vi "Size of Data from TD__ogtk.vi"(8 "error in":errorcluster, 10 "Type Descriptor":T1) -> (0 "error out":errorcluster, 2 "Size of Data":i32)   [LabVIEW 2011]
doc: "Returns the size of data of the TD. \nThe VI will return the following bytes of the listed datatypes:\n<b>1 byte</b> - I8, U8, Enum U8, Boolean\n<b>2 bytes</b> - 16, U16, Enum U16 \n<b>4 bytes</b> - I32, U32, SGL, Enum U32, Refnum\n<b>8 bytes</b> - I64, U64, DBL, CSG, Enum U64 \n<b>16 bytes</b> - EXT, CDB\n<b>32 bytes</b> - CXT\n<b>-1</b> - String, Path, Array \n<b>Sum of Bytes</b> - Cluster, VI calls itself recursively"
uses:
  Type Descriptor__ogtk.ctl
panel:
  in  "for recursive call to self":refnum<vi>
  # "[OpenG VI Tags] ***Do Not Remove***"
  # "Size of Data from TD.vi\n\nReturns the data size of the type defined by the TD.  This vi calls itself recurs\n\nPlease visit http://www.OpenG.org to learn about the\nOpen Source LabVIEW software movement.\n\nNOTICE -- YOU MUST LEAVE THIS NOTICE IN PLACE.  PER THE TERMS OF THE LICENSE BELOW, YOU MAY SUBLICENSE THIS SOFTWARE \nIN ANY WAY THAT DOES NOT CONFLICT WITH THIS LICENSE.\n\n### BSD License (http://www.opensource.org/licenses/bsd-license.php) Begin ###\n \nCopyright (c) 2002, Jean-Pierre Drolet <drolet_jp@hotmail.com>\nCopyright (c) 2002-2006, Jim Kring <jim@jimkring.com>\n\nAll rights reserved.\n\nRedistribution and use in source and binary forms, with or without modification, are permitted provided that the following conditions are met:\n\n    * Redistributions of source code must retain the above copyright notice, this list of conditions and the following disclaimer.\n    * Redistributions in binary form must reproduce the above copyright notice, this list of conditions and the following disclaimer in the \n       documentation and/or other materials provided with the distribution.\n    * Neither the name of SciWare, James Kring, Inc., nor the names of its contributors may be used to endorse or promote products derived \n       from this software without specific prior written permission.\n\nTHIS SOFTWARE IS PROVIDED BY THE COPYRIGHT HOLDERS AND CONTRIBUTORS \"AS IS\" AND ANY EXPRESS OR IMPLIED WARRANTIES, \nINCLUDING, BUT NOT LIMITED TO, THE IMPLIED WARRANTIES OF MERCHANTABILITY AND FITNESS FOR A PARTICULAR PURPOSE ARE \nDISCLAIMED. IN NO EVENT SHALL THE COPYRIGHT OWNER OR CONTRIBUTORS BE LIABLE FOR ANY DIRECT, INDIRECT, INCIDENTAL,\n SPECIAL, EXEMPLARY, OR CONSEQUENTIAL DAMAGES (INCLUDING, BUT NOT LIMITED TO, PROCUREMENT OF SUBSTITUTE GOODS OR \nSERVICES; LOSS OF USE, DATA, OR PROFITS; OR BUSINESS INTERRUPTION) HOWEVER CAUSED AND ON ANY THEORY OF LIABILITY, \nWHETHER IN CONTRACT, STRICT LIABILITY, OR TORT (INCLUDING NEGLIGENCE OR OTHERWISE) ARISING IN ANY WAY OUT OF THE USE \nOF THIS SOFTWARE, EVEN IF ADVISED OF THE POSSIBILITY OF SUCH DAMAGE.\n\n### BSD License End ###"
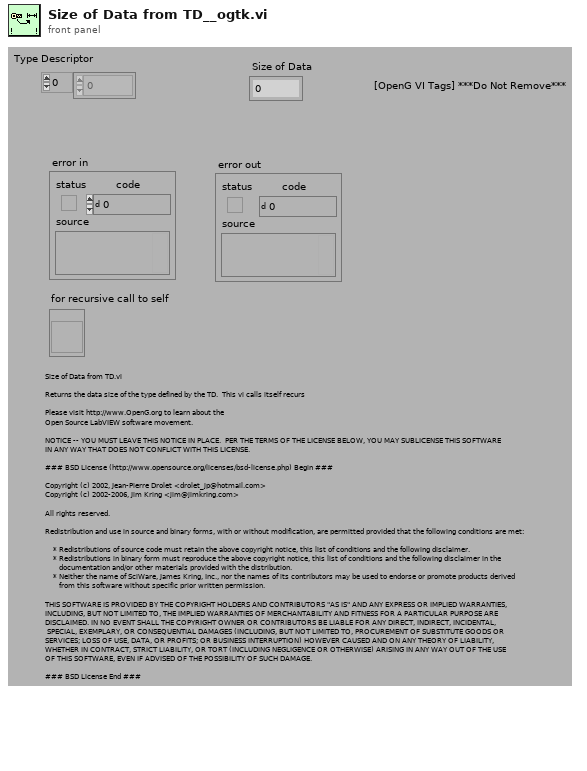
[diagram p1: front panel]
types:
  T1 = typedef "Type Descriptor__ogtk.ctl" = i16[]
  T2 = typedef "Type Descriptor Header__ogtk.ctl" = cluster{"length":u16, "private":u8, "type":T3, "# elements":u16}
  T3 = typedef "Type Descriptor Enumeration__ogtk.ctl" = enum8{"<Null>", "I8", "I16", "I32", "I64", "U8", "U16", "U32", "U64", "SGL", "DBL", "EXT", "CSG", "CDB", "CXT", "0x0F", "0x10", "0x11", "0x12", "0x13", "0x14", "Enum U8", "Enum U16", "Enum U32", "Enum U64", "SGL PQ", "DBL PQ", "EXT PQ", "CSG PQ", "CDB PQ", "CXT PQ", "0x1F", "0x20", "Boolean", "0x22", "0x23", "0x24", "0x25", "0x26", "0x27", "0x28", "0x29", "0x2A", "0x2B", "0x2C", "0x2D", "0x2E", "0x2F", "String", "0x31", "Path", "Pict", "0x34", "0x35", "0x36", "DAQ", "0x38", "0x39", "0x3A", "0x3B", "0x3C", "0x3D", "0x3E", "0x3F", "Array", "0x41", "0x42", "0x43", "0x44", "0x45", "0x46", "0x47", "0x48", "0x49", "0x4A", "0x4B", "0x4C", "0x4D", "0x4E", "0x4F", "Cluster", "0x51", "0x52", "Variant", "Waveform", "0x55", "0x56", "0x57", "0x58", "0x59", "0x5A", "0x5B", "0x5C", "0x5D", "0x5E", "0x5F", "0x60", "0x61", "0x62", "0x63", "0x64", "0x65", "0x66", "0x67", "0x68", "0x69", "0x6A", "0x6B", "0x6C", "0x6D", "0x6E", "0x6F", "Refnum"}
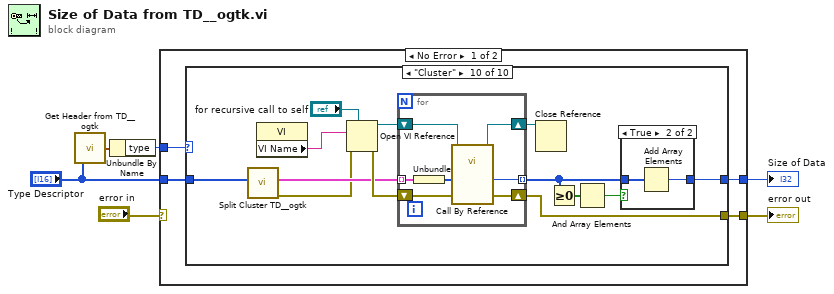
[diagram p0: block diagram]
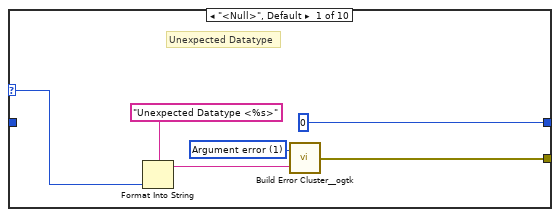
[diagram p2: hidden frame]
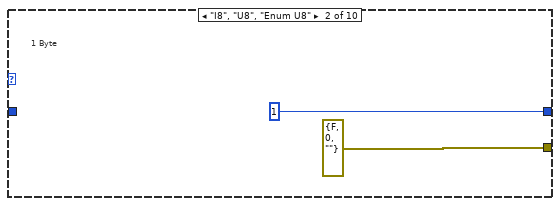
[diagram p3: hidden frame]
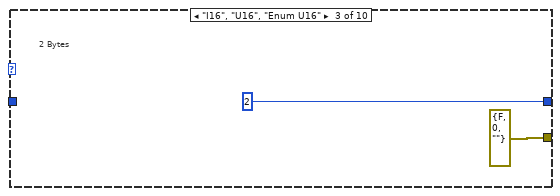
[diagram p4: hidden frame]
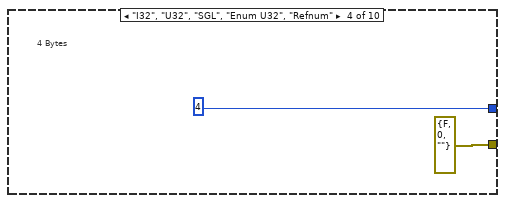
[diagram p5: hidden frame]
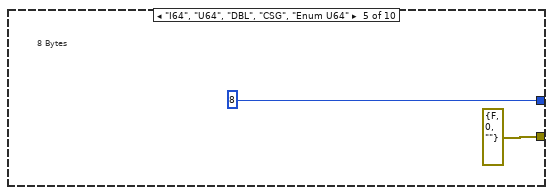
[diagram p6: hidden frame]
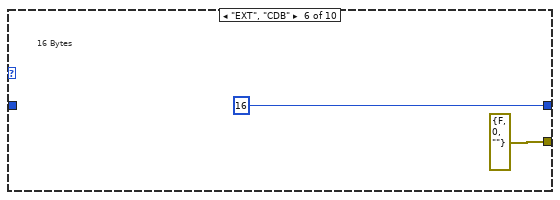
[diagram p7: hidden frame]
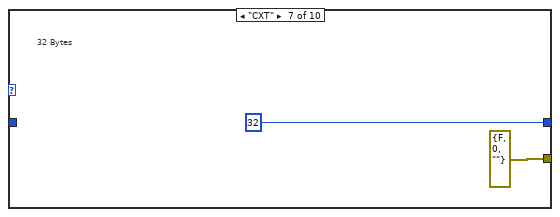
[diagram p8: hidden frame]
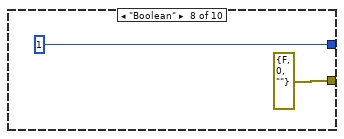
[diagram p9: hidden frame]
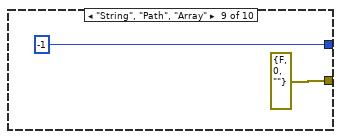
[diagram p10: hidden frame]
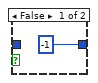
[diagram p11: hidden frame]
diagram:
  n1 = call "Get Header from TD__ogtk.vi"("Type Descriptor"="Type Descriptor") -> ("Type Descriptor Header"=w2:T2)
  n2 = Unbundle By Name(w2) -> ("type"=w1:T3)
  n3 = case shown="No Error" "error in" {
    selector: "error in" -> [_ w57]
    tunnel: w1 -> [w10 _]
    tunnel: [w9 w57] -> w4
    tunnel: "Type Descriptor" -> [w8 _]
    tunnel: [w7 0 ("Size of Data")] -> w3
    frame No Error {
      n4 = case shown="\"Cluster\"" w10 {
        selector: w10 -> [w13 _ _ _ _ _ _ _ _ _]
        tunnel: [w12 errorcluster {"status"=FALSE, "code"=0, "source"=""} ("error out") errorcluster {"status"=FALSE, "code"=0, "source"=""} ("error out") errorcluster {"status"=FALSE, "code"=0, "source"=""} ("error out") errorcluster {"status"=FALSE, "code"=0, "source"=""} ("error out") errorcluster {"status"=FALSE, "code"=0, "source"=""} ("error out") errorcluster {"status"=FALSE, "code"=0, "source"=""} ("error out") errorcluster {"status"=FALSE, "code"=0, "source"=""} ("error out") errorcluster {"status"=FALSE, "code"=0, "source"=""} ("error out") w36] -> w9
        tunnel: w8 -> [_ _ _ _ _ _ _ _ _ w35]
        tunnel: [0 ("Size of Data") 1 2 4 8 16 32 1 -1 w37] -> w7
        frame "<Null>", Default {
          w14 = 1 items=["No error", "Argument error", "Memory is full", "Out of zone", "End of file", "File already open", "Generic file I/O error", "File not found", "File permission error", "Disk is full", "Duplicate path", "Too many files open", "System feature not enabled", "Resource file not found", "Cannot add resource", "Resource not found", "Image not found", "Image memory error", "Pen does not exist", "Config type invalid", "Config token not found", "Config parse error", "Config memory error", "Bad external code format", "Bad external code offset", "External code not present", "Null window", "Destroy window error", "Null menu", "Print aborted", "Bad print record", "Print driver error", "Windows error during printing", "Memory error during printing", "Print dialog error", "Generic print error", "Invalid device refnum", "Device not found", "Device parameter error", "Device unit error", "Cannot open device", "Device call aborted", "Generic error", "Cancelled by user", "Object ID too low", "Object ID too high", "Object not in heap", "Unknown heap", "Unknown object (invalid DefProc)", "Unknown object (DefProc not in table)", "Message out of range", "Invalid (null) method", "Unknown message", "Manager call not supported", "Bad address", "Network operation in progress", "Network operation timed out", "Connection is busy", "Network attribute not supported", "Network error", "Address in use", "System out of memory", "Connection aborted", "Connection refused", "Not connected", "Already connected", "Connection closed", "Initialization error (interapplication manager)", "Bad occurrence", "Wait on unbound occurrence handler", "Occurrence queue overflow", "Datalog type conflict", "Unused", "Unrecognized type (interapplication manager)", "Memory corrupt", "Failed to make temporary DLL", "Old CIN version", "Drag socket not found", "Failed to load drop-object", "Failed to register OLE object", "Failed to release OLE object", "Format specifier type mismatch", "Unknown format specifier", "Too few format specifiers", "Too many format specifiers", "Scan failed", "Newer CIN version", "Error converting to variant", "Runtime menu error", "Password tampered", "Variant attribute not found", "Incompatible variant data type", "Event data is not available", "Event Store is not present", "Occurrence is not found", "Event Queue is not created", "Event info is not available", "Refnum passed is NULL", "Error retrieving Class GUID", "Error retrieving CoClass GUID", "Error retrieving TypeLib GUID.", "Bad built application magic bytes.", "Specific driver is different from the specific driver associated with the Logical Name.", "There is no session opened to the class driver.", "Max Error", "MAX - Error with config objects", "MAX - Error loading configuration", "MAX - Group not supported"]
          # "Unexpected Datatype"
          n5 = Format Into String(format string="Unexpected Datatype <%s>" ("Format String"), w13) -> (resulting string=w16:string)  [unwired: 2 in, 1 out]
          n6 = call "Build Error Cluster__ogtk.vi"("String to Prepend to source (\"\")"=w16, "code"=w14) -> ("error out"=w12:errorcluster)
        }
        frame "I8", "U8", "Enum U8" {
          # "1 Byte"
        }
        frame "I16", "U16", "Enum U16" {
          # "2 Bytes"
        }
        frame "I32", "U32", "SGL", "Enum U32", "Refnum" {
          # "4 Bytes"
        }
        frame "I64", "U64", "DBL", "CSG", "Enum U64" {
          # "8 Bytes"
        }
        frame "EXT", "CDB" {
          # "16 Bytes"
        }
        frame "CXT" {
          # "32 Bytes"
        }
        frame "Boolean" {
        }
        frame "String", "Path", "Array" {
        }
        frame "Cluster" {
          n7 = call "Split Cluster TD__ogtk.vi"("Type Descriptor"=w35) -> ("error out"=w33:errorcluster, "Type Descriptors"=w34:cluster{"Type Descriptor":T1}[])  [unwired: 9 in]
          n8 = property class="VI"() -> ("VI Name"=w45:string)  [unwired: 2 in, 2 out]
          n9 = Open VI Reference(type specifier VI Refnum (for type only)="for recursive call to self", vi path=w45, error in (no error)=w33) -> (vi reference=w43:refnum<vi>, error out=w42:errorcluster)  [unwired: 3 in]
          n10 = for {
            tunnel: w34 -> [w55] mode=indexing
            shift-right: [w49] -> w36
            shift-left: w42 -> [w50]
            shift-right: [w53] -> w41
            shift-left: w43 -> [w54]
            tunnel: [w51] -> w38 mode=indexing
            n11 = Unbundle(w55) -> ("Type Descriptor"=w52:T1)
            n12 = call-by-ref "?"(reference=w54, "error in"=w50, "type string"=w52) -> (reference out=w53:refnum<vi>, "error out"=w49:errorcluster, "Size of Data"=w51:i32)  [unwired: 9 in, 1 out]
          }
          n13 = Close Reference(reference=w41) -> ()  [unwired: 1 in, 1 out]
          n14 = Greater Or Equal To 0?(x=w38) -> (x >= 0?=w40:bool[])
          n15 = And Array Elements(Boolean array=w40) -> (logical AND=w39:bool)
          n16 = case shown="True" w39 {
            tunnel: w38 -> [_ w48]
            tunnel: [-1 ("Size of Data") w47] -> w37
            frame False {
            }
            frame True {
              n17 = Add Array Elements(numeric array=w48) -> (sum=w47:i32)
            }
          }
        }
      }
    }
    frame Error {
    }
  }
  "error out" <- w4
  "Size of Data" <- w3
